vi "PXI_Host_Cluster_Read_OldMethod_Benchmark.vi"() -> ()   [LabVIEW 2018]
uses:
  cRIO RT/TypeDefs/Simple cluster.ctl
  <vilib>/addons/FPGA Advanced Session Resources/LVFPGA Adv Session Resources/OpenByNameSubVI.vi
  <vilib>/rvi/interface/common/dynamic/niFpgaEscapeDelimiterAndNull.vi
  <vilib>/Utility/error.llb/Error Cluster From Error Code.vi
  <vilib>/rvi/errors/niLvFpgaAdjustHostInterfaceError.vi
  <vilib>/FPGAPlugInAG/Dynamic/niLvFpga_Close_Dynamic.vi
  <vilib>/addons/FPGA Advanced Session Resources/LVFPGA Adv Session Resources/OpenByName.xnode
  <vilib>/rvi/interface/nirviReadWriteControl/nirviReadWriteControl.xnode
  <vilib>/rvi/interface/nirviCloseFPGA/nirviCloseFPGA.xnode
  NiFpgaLv.dll
  <vilib>/rvi/interface/Simulation/niFpgaSimulationCallBeginRW.vi
  <vilib>/addons/FPGA Advanced Session Resources/LVFPGA Adv Session Resources/LVFPGAAdvSessionResources.lvlib
panel:
  out "Value":T1
  out "error out":errorcluster
  out "Execution time (s)":dbl
  # "Recorded time"
  # "3.37551E-5"
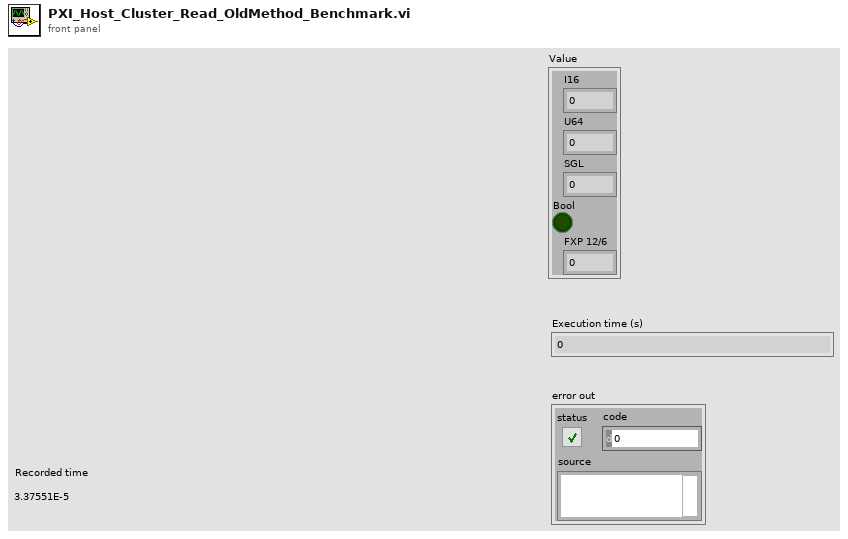
[diagram p1: front panel]
types:
  T1 = cluster{"I16":i16, "U64":u64, "SGL":sgl, "Bool":bool, "FXP 12/6":fxp<+/-,12,6>}
  T2 = typedef "Simple cluster.ctl" = cluster{"I16":i16, "U64":u64, "SGL":sgl, "Bool":bool, "FXP 12/6":fxp<+/-,12,6>}
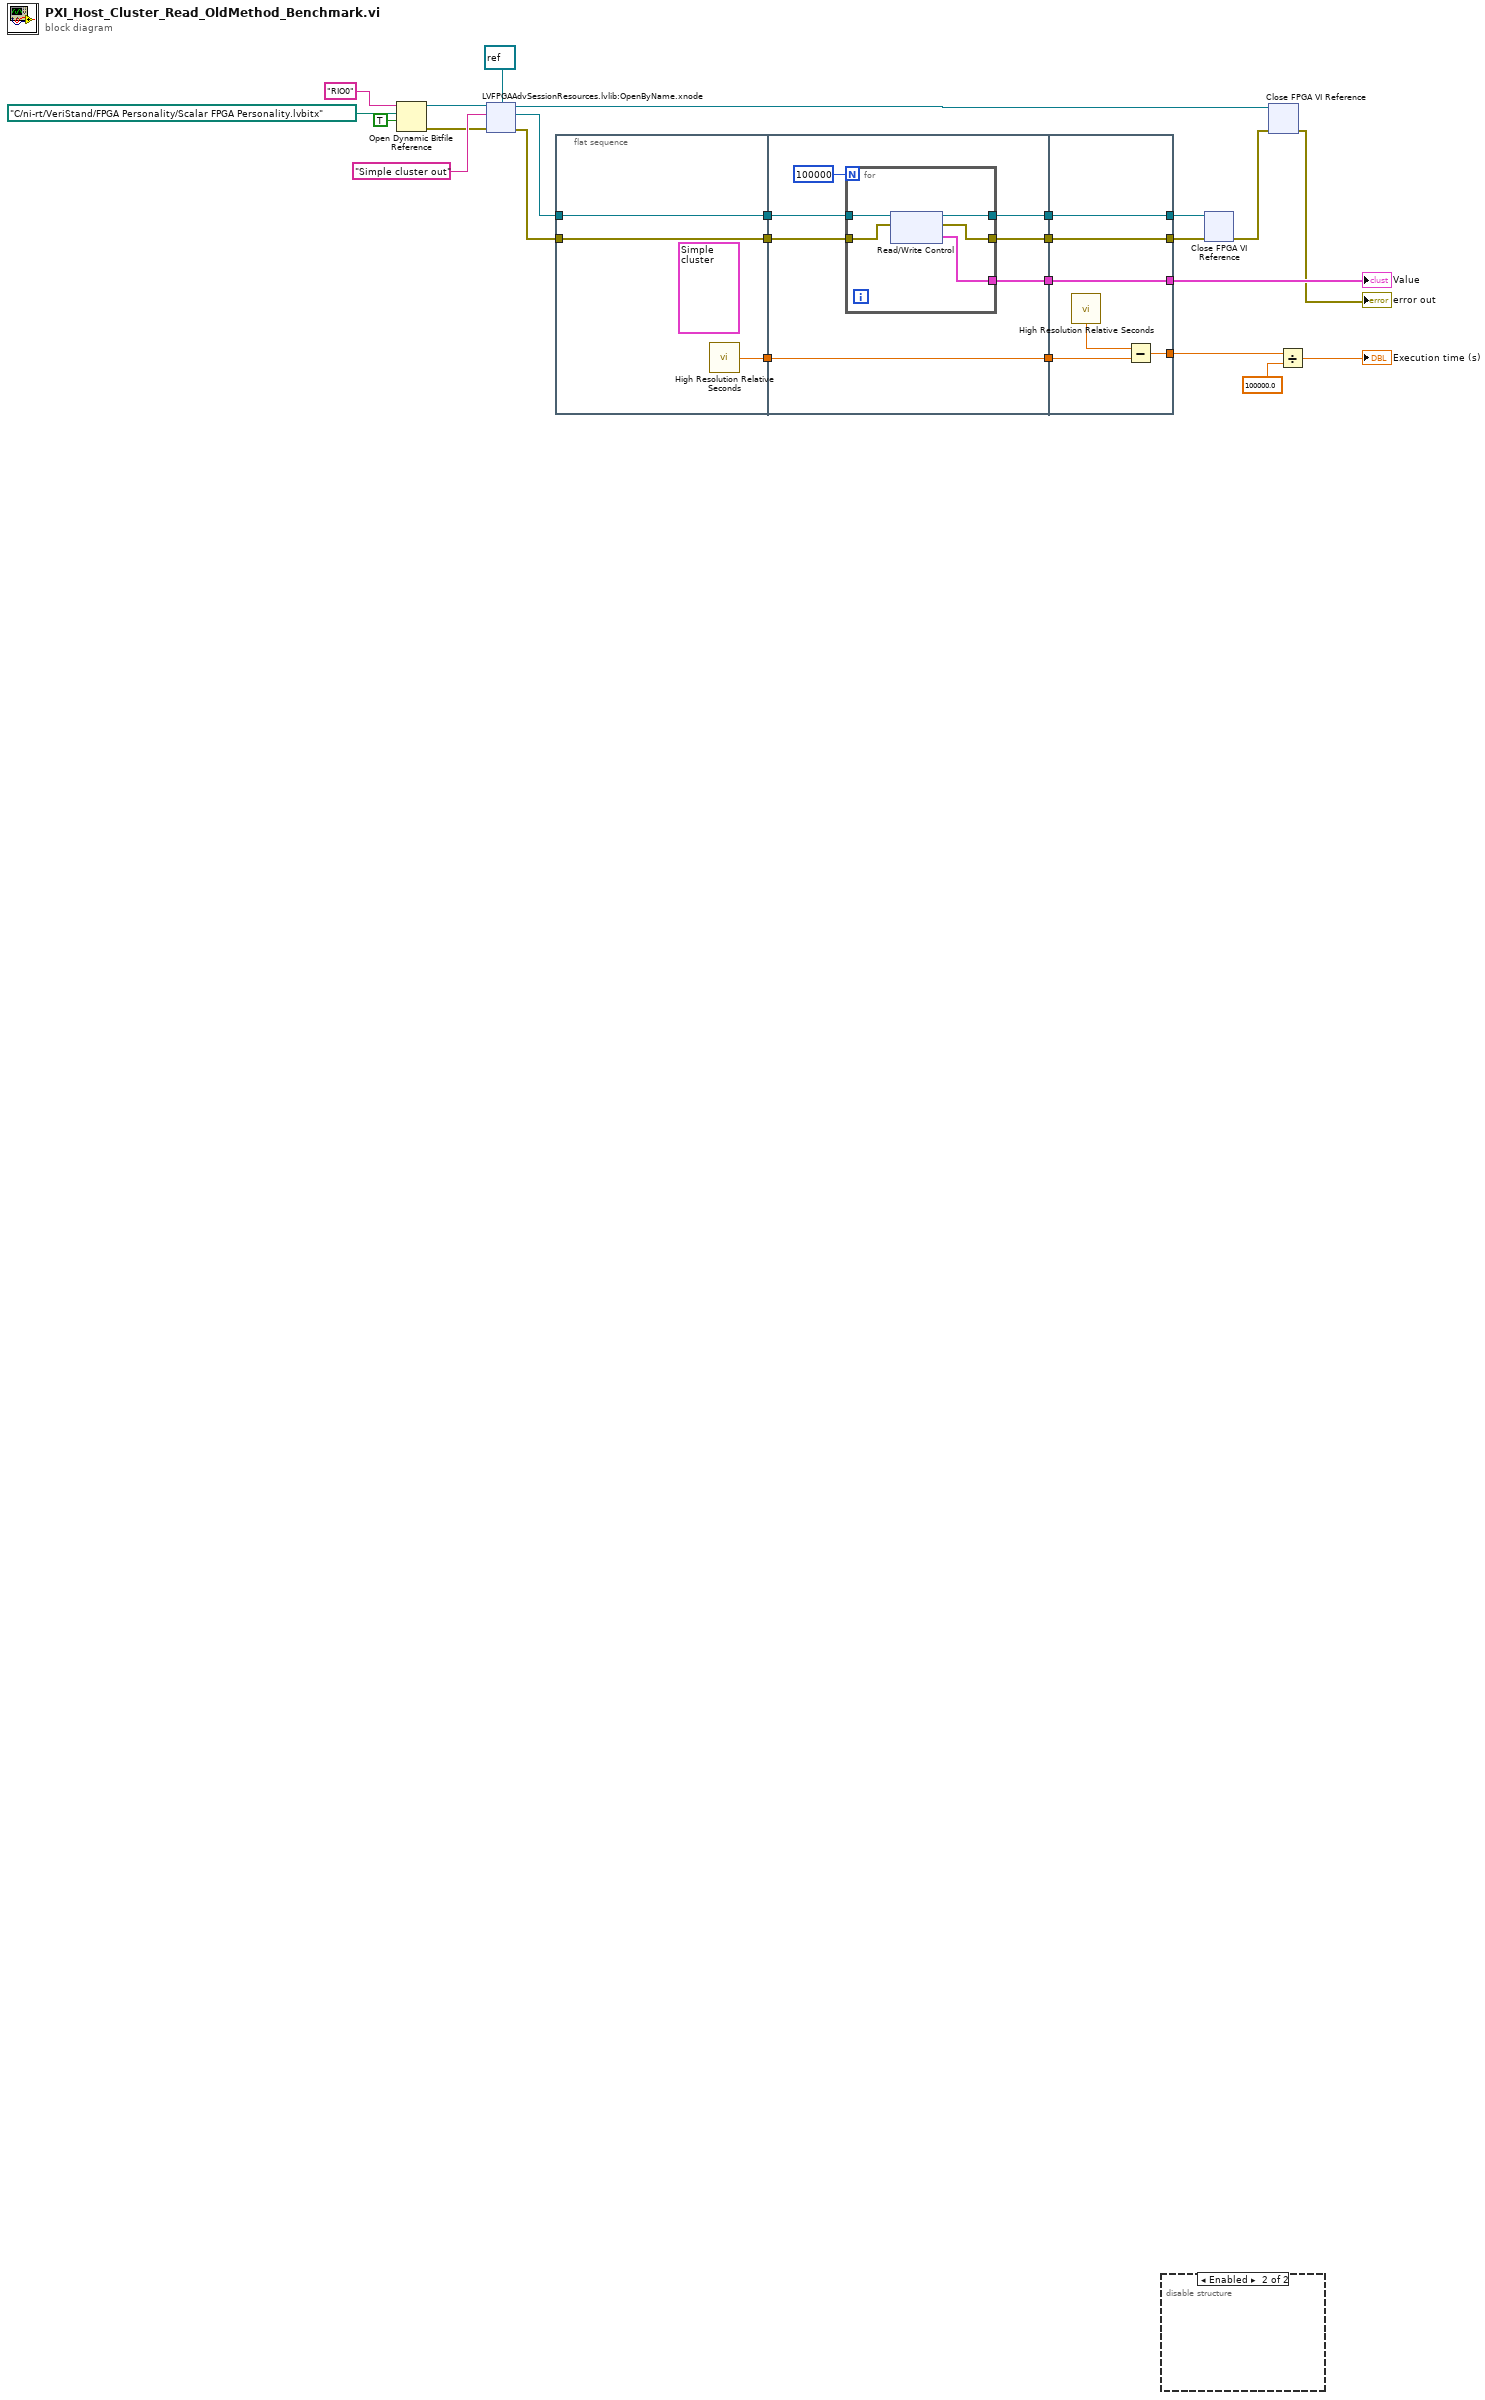
[diagram p0: block diagram]
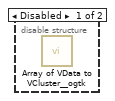
[diagram p2: hidden frame]
diagram:
  n1 = Open Dynamic Bitfile Reference(0:"RIO0" ("Device address"), 1:path "C:/ni-rt/VeriStand/FPGA Personality/Scalar FPGA Personality.lvbitx" ("Bitfile path"), 2:TRUE ("Run When Loaded")) -> (5:w11:refnum<k20>, 8:w9:errorcluster)  [unwired: 2 in]
  n2 = xnode "LVFPGAAdvSessionResources.lvlib:OpenByName.xnode"("FPGA VI Reference in"=w11, "Resource name in"="Simple cluster out", "Single resource reference type in"=refnum<k20> refnum ("Type"), "Error in"=w9) -> ("Single resource reference out"=w7:refnum<k20>, "Error out"=w8:errorcluster, "FPGA VI Reference out"=w3:refnum<k20>)
  n3 = flat-sequence {
    tunnel: [w28] -> w24
    tunnel: w7 -> [w27]
    tunnel: [w27] -> w17
    tunnel: [w26] -> w16
    tunnel: w8 -> [w26]
    tunnel: [w34] -> w25
    tunnel: w24 -> [w34]
    tunnel: w17 -> [w33]
    tunnel: w16 -> [w32]
    tunnel: [w31] -> w15
    tunnel: [w30] -> w14
    tunnel: [w29] -> w5
    tunnel: w25 -> [w45]
    tunnel: [w44] -> w23
    tunnel: w15 -> [w42]
    tunnel: w14 -> [w43]
    tunnel: [w43] -> w13
    tunnel: [w42] -> w12
    tunnel: [w41] -> w4
    tunnel: w5 -> [w41]
    frame #0 {
      (unwired) T2 {"I16"=1231, "U64"=213123, "SGL"=1.0, "Bool"=TRUE, "FXP 12/6"=31.984375} ("Simple Cluster")
      n4 = call <vilib>:"High Resolution Relative Seconds.vi"() -> ("relative seconds"=w28:dbl)
    }
    frame #1 {
      n5 = for {
        N: 100000 -> [_]
        tunnel: w33 -> [w40]
        tunnel: w32 -> [w39]
        tunnel: [w38] -> w31
        tunnel: [w37] -> w30
        tunnel: [w36] -> w29
        n6 = xnode "Read/Write Control"("FPGA VI Reference In"=w40, "error in"=w39) -> ("FPGA VI Reference Out"=w37:refnum<k20>, "error out"=w38:errorcluster, "Value"=w36:T1)
      }
    }
    frame #2 {
      n7 = call <vilib>:"High Resolution Relative Seconds.vi"() -> ("relative seconds"=w46:dbl)
      n8 = Subtract(x=w46, y=w45) -> (x-y=w44:dbl)
    }
  }
  n9 = disable-structure shown="Enabled" {
    frame Disabled {
      n10 = call <userlib>:"Array of VData to VCluster__ogtk.vi"() -> ()  [unwired: 10 in, 2 out]
    }
    frame Enabled {
    }
  }
  n11 = xnode "Close FPGA VI Reference"("FPGA VI Reference In"=w13, "error in"=w12) -> ("error out"=w2:errorcluster)
  n12 = xnode "Close FPGA VI Reference"("FPGA VI Reference In"=w3, "error in"=w2) -> ("error out"=→"error out":errorcluster)
  n13 = Divide(x=w23, y=100000.0) -> (x/y=→"Execution time (s)":dbl)
  "Value" <- w4
